vi "Global Connection Engine.vi"(5 "Receiver Data Type":T1, 6 "Connection Action":T2=enum."Get Connections", 7 "Receiver Channel In":variant, 9 "Signal Index":i32, 10 "LQObject Manifestation":u64) -> (2 "Receiver Channels Out":variant[](array[variant]))   [LabVIEW 2013, in "Template.lvlib" / "LQCoreEngine.lvclass"]
uses:
  LQCoreEngine.lvclass
  Connection Action.ctl
  Signal Data Type.ctl
  <vilib>/Utility/VariantDataType/VariantType.lvlib
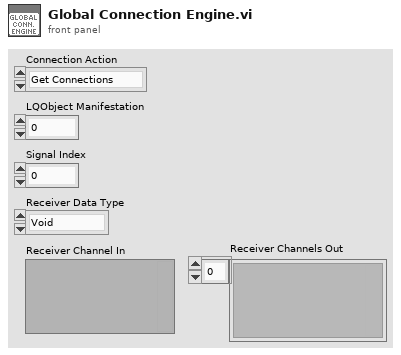
[diagram p1: front panel]
types:
  T1 = typedef "Template.lvlib/LQCoreEngine.lvclass/Signal Data Type.ctl" = enum16{"Void", "Bool", "I32", "DBL", "String"}
  T2 = typedef "Template.lvlib/LQCoreEngine.lvclass/Connection Action.ctl" = enum16{"Init", "Add Connection", "Get Connections", "Clean Up"}
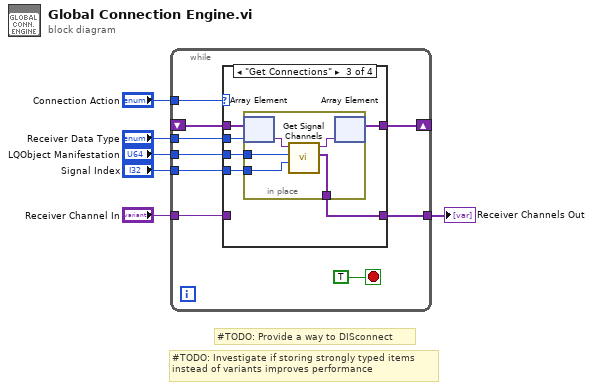
[diagram p0: block diagram]
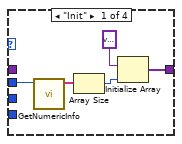
[diagram p2: hidden frame]
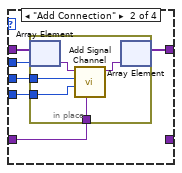
[diagram p3: hidden frame]
diagram:
  # "#TODO: Investigate if storing strongly typed items\ninstead of variants improves performance"
  # "#TODO: Provide a way to DISconnect"
  n1 = while {
    tunnel: "Connection Action" -> [w15]
    tunnel: "LQObject Manifestation" -> [w13]
    tunnel: "Signal Index" -> [w12]
    tunnel: "Receiver Channel In" -> [w11]
    tunnel: [w10] -> w2
    shift-right: [w9] -> _
    shift-left: _ -> [w8]
    tunnel: "Receiver Data Type" -> [w7]
    stop <- TRUE stop-if-true
    n2 = case shown="\"Get Connections\"" w15 {
      tunnel: w13 -> [_ w26 w37 _]
      tunnel: w12 -> [_ w25 w36 _]
      tunnel: w11 -> [_ w24 _ _]
      tunnel: [_ _ w35 _] -> w10
      tunnel: [w18 w21 w33 w43] -> w9
      tunnel: w8 -> [_ w23 w34 w43]
      tunnel: w7 -> [w16 w22 w32 _]
      frame "Init" {
        n3 = call <vilib>:"GetNumericInfo.vi"("Variant"=w16) -> ("EnumNames"=w20:string[])  [unwired: 7 in, 3 out]
        n4 = Array Size(array=w20) -> (size(s)=w19:i32)
        n5 = Initialize Array(variant ("Signal Map"), w19) -> (w18:variant[])
      }
      frame "Add Connection" {
        n6 = in-place {
          in-place-border: w26 -> [w31]
          in-place-border: w25 -> [w30]
          in-place-border: w24 -> [w29]
          n7 = in-place-array #1(w23, w22) -> (w28:variant)
          n8 = call "Add Signal Channel.vi"("Signal Channel"=w29, "Signal Index"=w30, "QObject Refnum"=w31, "Signal Map"=w28) -> ("Modified Signal Map"=w27:variant)  [unwired: 7 in]
          n9 = in-place-array #1(w27) -> (w21:variant[])  [unwired: 1 out]
        }
      }
      frame "Get Connections" {
        n10 = in-place {
          in-place-border: w37 -> [w42]
          in-place-border: w36 -> [w41]
          in-place-border: [w40] -> w35
          n11 = in-place-array #2(w34, w32) -> (w39:variant)
          n12 = call "Get Signal Channels.vi"("Signal Index"=w41, "LQObject Manifestation"=w42, "Signal Map"=w39) -> ("Signal Channels"=w40:variant[], "Dup. Signal Map"=w38:variant)  [unwired: 7 in]
          n13 = in-place-array #2(w38) -> (w33:variant[])  [unwired: 1 out]
        }
      }
      frame "Clean Up" {
        # "#TODO: Clean up"
      }
    }
  }
  "Receiver Channels Out" <- w2
